vi "S4GUI.vi"(7 "Tab ObsEng":enum32{"Obs", "CCD modes", "Eng"}(tab)) -> ()   [LabVIEW 2018] (continued)
                n2324 = call "Write Exposure Time.vi"("error in (no error)"=w4861, "Exposure Time"=w4839, "Interface in"=w4872) -> ("error out"=w4840:errorcluster, "Interface out"=w4841:refnum<class "Interface.lvclass">)  [unwired: 7 in]
                n2325 = case shown="Default" w4838 {
                  tunnel: w4841 -> [w4887 w4892]
                  tunnel: [w4887 w4891] -> w4837
                  tunnel: [w4886 w4890] -> w4836
                  tunnel: w4840 -> [w4886 w4889]
                  tunnel: w4839 -> [_ w4888]
                  frame "ZERO" {
                  }
                  frame Default {
                    n2326 = call-dynamic "Write prev ExpTime.vi"("error in (no error)"=w4889, "prev ExpTime"=w4888, "Interface in"=w4892) -> ("error out"=w4890:errorcluster, "Interface out"=w4891:refnum<class "Interface.lvclass">)  [unwired: 7 in]
                  }
                }
                n2327 = call-dynamic "Write Suffix.vi"("error in (no error)"=w4836, "Suffix"=w4881, "Interface in"=w4837) -> ("error out"=w4862:errorcluster, "Interface out"=w4873:refnum<class "Interface.lvclass">)  [unwired: 7 in]
                n2328 = call-dynamic "Write ObsType.vi"("error in (no error)"=w4862, "ObsType"=w4856, "Interface in"=w4873) -> ("error out"=w4863:errorcluster, "Interface out"=w4874:refnum<class "Interface.lvclass">)  [unwired: 7 in]
                n2329 = call-dynamic "Write Object.vi"("error in (no error)"=w4863, "Object"=w4855, "Interface in"=w4874) -> ("error out"=w4864:errorcluster, "Interface out"=w4875:refnum<class "Interface.lvclass">)  [unwired: 7 in]
                n2330 = call-dynamic "Write Comments.vi"("error in (no error)"=w4864, "Comments"=w4880, "Interface in"=w4875) -> ("error out"=w4865:errorcluster, "Interface out"=w4876:refnum<class "Interface.lvclass">)  [unwired: 7 in]
                n2331 = local read "Exp ch2"() -> (w4859:u32)
                n2332 = call-dynamic "Write DS9.vi"("error in (no error)"=w4865, "DS9"="F", "Interface in"=w4876) -> ("error out"=w4852:errorcluster, "Interface out"=w4854:refnum<class "Interface.lvclass">)  [unwired: 7 in]
                n2333 = call-dynamic "Write Observer.vi"("error in (no error)"=w4852, "Observer"=w4850, "Interface in"=w4854) -> ("error out"=w4851:errorcluster, "Interface out"=w4853:refnum<class "Interface.lvclass">)  [unwired: 7 in]
                n2334 = call-dynamic "Write # Images.vi"("error in (no error)"=w4851, "# Images"=w4859, "Interface in"=w4853) -> ("error out"=w4866:errorcluster, "Interface out"=w4877:refnum<class "Interface.lvclass">)  [unwired: 7 in]
                n2335 = property on="Exposure Time ch2" class="Slide (strict)"("Scale.Maximum"=w4839, "Scale.Minimum"=0.0 ("Scale.Range:Minimum")) -> ()  [unwired: 2 in, 2 out]
                n2336 = property on="Exposures Done ch2" class="Slide (strict)"("Scale.Maximum"=w4859, "Scale.Minimum"=0.0 ("Scale.Range:Minimum")) -> ()  [unwired: 2 in, 2 out]
                n2337 = call-dynamic "Write Interface.vi"("error in (no error)"=w4866, "Interface.lvclass"=w4877, "Channel in"=w4871) -> ("error out"=w4849:errorcluster, "Channel out"=w4848:refnum<class "Channel.lvclass">)  [unwired: 7 in]
                n2338 = call-dynamic "Write ciclos.vi"("error in (no error)"=w4849, "ciclos"=w4847, "Channel in"=w4848) -> ("error out"=w4844:errorcluster, "Channel out"=w4846:refnum<class "Channel.lvclass">)  [unwired: 7 in]
                n2339 = call-dynamic "Write sequencias.vi"("error in (no error)"=w4844, "sequencias"=w4842, "Channel in"=w4846) -> ("error out"=w4843:errorcluster, "Channel out"=w4845:refnum<class "Channel.lvclass">)  [unwired: 7 in]
                n2340 = call-dynamic "Write Channel.vi"("error in (no error)"=w4843, "Channel.lvclass"=w4845, "Acquisition in"=w4879) -> ("error out"=w4833:errorcluster, "Acquisition out"=w4835:refnum<class "Acquisition.lvclass">)  [unwired: 7 in]
                n2341 = call-dynamic "CalcCubeDuration.vi"("error in (no error)"=w4833, "Acquisition in"=w4835) -> ("error out"=w4832:errorcluster, "Acquisition out"=w4834:refnum<class "Acquisition.lvclass">)  [unwired: 8 in]
                n2342 = call "Write AcquisitionB.vi"("error in (no error)"=w4832, "Acquisition.lvclass"=w4834, "S4ACS_GUI in"=w4878) -> ("error out"=w4882:errorcluster, "S4ACS_GUI out"=w4883:refnum<class "S4GUI.lvclass">)  [unwired: 7 in]
              }
              frame #2 {
                # "object"
                # "suffix"
                # "obsType"
                n2343 = call-dynamic "Read AcquisitionC.vi"("error in (no error)"=w4945, "S4ACS_GUI in"=w4946) -> ("error out"=w4935:errorcluster, "Acquisition.lvclass"=w4934:refnum<class "Acquisition.lvclass">, "S4ACS_GUI out"=w4924:refnum<class "S4GUI.lvclass">)  [unwired: 7 in]
                n2344 = call-dynamic "Read Channel.vi"("error in (no error)"=w4935, "Acquisition in"=w4934) -> ("error out"=w4932:errorcluster, "Channel.lvclass"=w4933:refnum<class "Channel.lvclass">, "Acquisition out"=w4923:refnum<class "Acquisition.lvclass">)  [unwired: 7 in]
                n2345 = local read "Exptime ch3"() -> (w4900:dbl)
                n2346 = call-dynamic "Read Interface.vi"("error in (no error)"=w4932, "Channel in"=w4933) -> ("error out"=w4941:errorcluster, "Interface.lvclass"=w4930:refnum<class "Interface.lvclass">, "Channel out"=w4931:refnum<class "Channel.lvclass">)  [unwired: 7 in]
                n2347 = call "Write Exposure Time.vi"("error in (no error)"=w4941, "Exposure Time"=w4900, "Interface in"=w4930) -> ("error out"=w4901:errorcluster, "Interface out"=w4902:refnum<class "Interface.lvclass">)  [unwired: 7 in]
                n2348 = case shown="\"ZERO\"" w4899 {
                  tunnel: w4902 -> [w4948 w4953]
                  tunnel: [w4948 w4952] -> w4898
                  tunnel: [w4947 w4951] -> w4897
                  tunnel: w4901 -> [w4947 w4950]
                  tunnel: w4900 -> [_ w4949]
                  frame "ZERO" {
                  }
                  frame Default {
                    n2349 = call-dynamic "Write prev ExpTime.vi"("error in (no error)"=w4950, "prev ExpTime"=w4949, "Interface in"=w4953) -> ("error out"=w4951:errorcluster, "Interface out"=w4952:refnum<class "Interface.lvclass">)  [unwired: 7 in]
                  }
                }
                n2350 = call-dynamic "Write Suffix.vi"("error in (no error)"=w4897, "Suffix"=w4942, "Interface in"=w4898) -> ("error out"=w4940:errorcluster, "Interface out"=w4929:refnum<class "Interface.lvclass">)  [unwired: 7 in]
                n2351 = call-dynamic "Write ObsType.vi"("error in (no error)"=w4940, "ObsType"=w4917, "Interface in"=w4929) -> ("error out"=w4939:errorcluster, "Interface out"=w4928:refnum<class "Interface.lvclass">)  [unwired: 7 in]
                n2352 = call-dynamic "Write Object.vi"("error in (no error)"=w4939, "Object"=w4916, "Interface in"=w4928) -> ("error out"=w4938:errorcluster, "Interface out"=w4927:refnum<class "Interface.lvclass">)  [unwired: 7 in]
                n2353 = call-dynamic "Write Comments.vi"("error in (no error)"=w4938, "Comments"=w4918, "Interface in"=w4927) -> ("error out"=w4937:errorcluster, "Interface out"=w4926:refnum<class "Interface.lvclass">)  [unwired: 7 in]
                n2354 = call-dynamic "Write DS9.vi"("error in (no error)"=w4937, "DS9"="F", "Interface in"=w4926) -> ("error out"=w4913:errorcluster, "Interface out"=w4915:refnum<class "Interface.lvclass">)  [unwired: 7 in]
                n2355 = local read "Exp ch3"() -> (w4921:u32)
                n2356 = property on="Exposure Time ch3" class="Slide (strict)"("Scale.Maximum"=w4900, "Scale.Minimum"=0.0 ("Scale.Range:Minimum")) -> ()  [unwired: 2 in, 2 out]
                n2357 = call-dynamic "Write Observer.vi"("error in (no error)"=w4913, "Observer"=w4911, "Interface in"=w4915) -> ("error out"=w4912:errorcluster, "Interface out"=w4914:refnum<class "Interface.lvclass">)  [unwired: 7 in]
                n2358 = property on="Exposures Done ch3" class="Slide (strict)"("Scale.Maximum"=w4921, "Scale.Minimum"=0.0 ("Scale.Range:Minimum")) -> ()  [unwired: 2 in, 2 out]
                n2359 = call-dynamic "Write # Images.vi"("error in (no error)"=w4912, "# Images"=w4921, "Interface in"=w4914) -> ("error out"=w4936:errorcluster, "Interface out"=w4925:refnum<class "Interface.lvclass">)  [unwired: 7 in]
                n2360 = call-dynamic "Write Interface.vi"("error in (no error)"=w4936, "Interface.lvclass"=w4925, "Channel in"=w4931) -> ("error out"=w4910:errorcluster, "Channel out"=w4909:refnum<class "Channel.lvclass">)  [unwired: 7 in]
                n2361 = call-dynamic "Write ciclos.vi"("error in (no error)"=w4910, "ciclos"=w4908, "Channel in"=w4909) -> ("error out"=w4905:errorcluster, "Channel out"=w4907:refnum<class "Channel.lvclass">)  [unwired: 7 in]
                n2362 = call-dynamic "Write sequencias.vi"("error in (no error)"=w4905, "sequencias"=w4903, "Channel in"=w4907) -> ("error out"=w4904:errorcluster, "Channel out"=w4906:refnum<class "Channel.lvclass">)  [unwired: 7 in]
                n2363 = call-dynamic "Write Channel.vi"("error in (no error)"=w4904, "Channel.lvclass"=w4906, "Acquisition in"=w4923) -> ("error out"=w4894:errorcluster, "Acquisition out"=w4896:refnum<class "Acquisition.lvclass">)  [unwired: 7 in]
                n2364 = call-dynamic "CalcCubeDuration.vi"("error in (no error)"=w4894, "Acquisition in"=w4896) -> ("error out"=w4893:errorcluster, "Acquisition out"=w4895:refnum<class "Acquisition.lvclass">)  [unwired: 8 in]
                n2365 = call-dynamic "Write AcquisitionC.vi"("error in (no error)"=w4893, "Acquisition.lvclass"=w4895, "S4ACS_GUI in"=w4924) -> ("error out"=w4943:errorcluster, "S4ACS_GUI out"=w4944:refnum<class "S4GUI.lvclass">)  [unwired: 7 in]
              }
              frame #3 {
                # "object"
                # "suffix"
                # "obsType"
                n2366 = call-dynamic "Read AcquisitionD.vi"("error in (no error)"=w5006, "S4ACS_GUI in"=w5007) -> ("error out"=w4996:errorcluster, "Acquisition.lvclass"=w4995:refnum<class "Acquisition.lvclass">, "S4ACS_GUI out"=w4985:refnum<class "S4GUI.lvclass">)  [unwired: 7 in]
                n2367 = local read "Exptime ch4"() -> (w4959:dbl)
                n2368 = call-dynamic "Read Channel.vi"("error in (no error)"=w4996, "Acquisition in"=w4995) -> ("error out"=w4993:errorcluster, "Channel.lvclass"=w4994:refnum<class "Channel.lvclass">, "Acquisition out"=w4984:refnum<class "Acquisition.lvclass">)  [unwired: 7 in]
                n2369 = call-dynamic "Read Interface.vi"("error in (no error)"=w4993, "Channel in"=w4994) -> ("error out"=w5002:errorcluster, "Interface.lvclass"=w4991:refnum<class "Interface.lvclass">, "Channel out"=w4992:refnum<class "Channel.lvclass">)  [unwired: 7 in]
                n2370 = call "Write Exposure Time.vi"("error in (no error)"=w5002, "Exposure Time"=w4959, "Interface in"=w4991) -> ("error out"=w4961:errorcluster, "Interface out"=w4963:refnum<class "Interface.lvclass">)  [unwired: 7 in]
                n2371 = case shown="Default" w4958 {
                  tunnel: w4963 -> [w5009 w5014]
                  tunnel: [w5009 w5013] -> w4962
                  tunnel: [w5008 w5012] -> w4960
                  tunnel: w4961 -> [w5008 w5011]
                  tunnel: w4959 -> [_ w5010]
                  frame "ZERO" {
                  }
                  frame Default {
                    n2372 = call-dynamic "Write prev ExpTime.vi"("error in (no error)"=w5011, "prev ExpTime"=w5010, "Interface in"=w5014) -> ("error out"=w5012:errorcluster, "Interface out"=w5013:refnum<class "Interface.lvclass">)  [unwired: 7 in]
                  }
                }
                n2373 = call-dynamic "Write Suffix.vi"("error in (no error)"=w4960, "Suffix"=w5003, "Interface in"=w4962) -> ("error out"=w5001:errorcluster, "Interface out"=w4990:refnum<class "Interface.lvclass">)  [unwired: 7 in]
                n2374 = call-dynamic "Write ObsType.vi"("error in (no error)"=w5001, "ObsType"=w4978, "Interface in"=w4990) -> ("error out"=w5000:errorcluster, "Interface out"=w4989:refnum<class "Interface.lvclass">)  [unwired: 7 in]
                n2375 = call-dynamic "Write Object.vi"("error in (no error)"=w5000, "Object"=w4977, "Interface in"=w4989) -> ("error out"=w4999:errorcluster, "Interface out"=w4988:refnum<class "Interface.lvclass">)  [unwired: 7 in]
                n2376 = call-dynamic "Write Comments.vi"("error in (no error)"=w4999, "Comments"=w4979, "Interface in"=w4988) -> ("error out"=w4998:errorcluster, "Interface out"=w4987:refnum<class "Interface.lvclass">)  [unwired: 7 in]
                n2377 = call-dynamic "Write DS9.vi"("error in (no error)"=w4998, "DS9"="F", "Interface in"=w4987) -> ("error out"=w4974:errorcluster, "Interface out"=w4976:refnum<class "Interface.lvclass">)  [unwired: 7 in]
                n2378 = property on="Exposure Time ch4" class="Slide (strict)"("Scale.Maximum"=w4959, "Scale.Minimum"=0.0 ("Scale.Range:Minimum")) -> ()  [unwired: 2 in, 2 out]
                n2379 = local read "Exp ch4"() -> (w4982:u32)
                n2380 = call-dynamic "Write Observer.vi"("error in (no error)"=w4974, "Observer"=w4972, "Interface in"=w4976) -> ("error out"=w4973:errorcluster, "Interface out"=w4975:refnum<class "Interface.lvclass">)  [unwired: 7 in]
                n2381 = property on="Exposures Done ch4" class="Slide (strict)"("Scale.Maximum"=w4982, "Scale.Minimum"=0.0 ("Scale.Range:Minimum")) -> ()  [unwired: 2 in, 2 out]
                n2382 = call-dynamic "Write # Images.vi"("error in (no error)"=w4973, "# Images"=w4982, "Interface in"=w4975) -> ("error out"=w4997:errorcluster, "Interface out"=w4986:refnum<class "Interface.lvclass">)  [unwired: 7 in]
                n2383 = call-dynamic "Write Interface.vi"("error in (no error)"=w4997, "Interface.lvclass"=w4986, "Channel in"=w4992) -> ("error out"=w4971:errorcluster, "Channel out"=w4970:refnum<class "Channel.lvclass">)  [unwired: 7 in]
                n2384 = call-dynamic "Write ciclos.vi"("error in (no error)"=w4971, "ciclos"=w4969, "Channel in"=w4970) -> ("error out"=w4967:errorcluster, "Channel out"=w4968:refnum<class "Channel.lvclass">)  [unwired: 7 in]
                n2385 = call-dynamic "Write sequencias.vi"("error in (no error)"=w4967, "sequencias"=w4964, "Channel in"=w4968) -> ("error out"=w4966:errorcluster, "Channel out"=w4965:refnum<class "Channel.lvclass">)  [unwired: 7 in]
                n2386 = call-dynamic "Write Channel.vi"("error in (no error)"=w4966, "Channel.lvclass"=w4965, "Acquisition in"=w4984) -> ("error out"=w4955:errorcluster, "Acquisition out"=w4957:refnum<class "Acquisition.lvclass">)  [unwired: 7 in]
                n2387 = call-dynamic "CalcCubeDuration.vi"("error in (no error)"=w4955, "Acquisition in"=w4957) -> ("error out"=w4954:errorcluster, "Acquisition out"=w4956:refnum<class "Acquisition.lvclass">)  [unwired: 8 in]
                n2388 = call-dynamic "Write AcquisitionD.vi"("error in (no error)"=w4954, "Acquisition.lvclass"=w4956, "S4ACS_GUI in"=w4985) -> ("error out"=w5004:errorcluster, "S4ACS_GUI out"=w5005:refnum<class "S4GUI.lvclass">)  [unwired: 7 in]
              }
            }
            n2389 = call-dynamic "Write sequencias.vi"("error in (no error)"=w4730, "sequencias"=w4726, "S4GUI in"=w4728) -> ("error out"=w4729:errorcluster, "S4GUI out"=w4727:refnum<class "S4GUI.lvclass">)  [unwired: 7 in]
            n2390 = call-dynamic "Write ciclos.vi"("error in (no error)"=w4729, "ciclos"=w4731, "S4ACS_GUI in"=w4727) -> ("error out"=w4733:errorcluster, "S4ACS_GUI out"=w4735:refnum<class "S4GUI.lvclass">)  [unwired: 7 in]
            n2391 = property on="#Cycles Done" class="Slide (strict)"("Scale.Maximum"=w4731, "Scale.Minimum"=0.0 ("Scale.Range:Minor Increment")) -> ()  [unwired: 2 in, 2 out]
            n2392 = call-dynamic "Write TotalCiclos.vi"("error in (no error)"=w4733, "TotalCiclos"=w4731, "S4GUI in"=w4735) -> ("error out"=w4732:errorcluster, "S4GUI out"=w4734:refnum<class "S4GUI.lvclass">)  [unwired: 7 in]
          }
        }
        n2393 = call-dynamic "Write User Event.vi"("error in (no error)"=w4567, "User Event"=w4564, "S4GUI in"=w4568) -> ("error out"=w4566:errorcluster, "S4GUI out"=w4565:refnum<class "S4GUI.lvclass">)  [unwired: 7 in]
        n2394 = property on="Pause SM" class="Bool"(error in=w4566, "DisabledEnum"=T12."Enabled" ("Disabled")) -> (error out=w4585:errorcluster)  [unwired: 1 in, 1 out]
      }
      event "# Cycles": Value Change {
        w5015 = 0.0 ("Scale.Range:Minor Increment")
        n2395 = event-data() -> ("NewVal"=w5016:u32)  [unwired: 1 in]
        n2396 = call-dynamic "Write ciclos.vi"("error in (no error)"=w5019, "ciclos"=w5016, "S4ACS_GUI in"=w5020) -> ("error out"=w5018:errorcluster, "S4ACS_GUI out"=w5017:refnum<class "S4GUI.lvclass">)  [unwired: 7 in]
        n2397 = property on="#Cycles Done" class="Slide (strict)"("Scale.Maximum"=w5016, "Scale.Minimum"=w5015) -> ()  [unwired: 2 in, 2 out]
        n2398 = property on="Cycles Done ch2" class="Slide (strict)"("Scale.Maximum"=w5016, "Scale.Minimum"=w5015) -> ()  [unwired: 2 in, 2 out]
        n2399 = property on="Cycles Done ch4" class="Slide (strict)"("Scale.Maximum"=w5016, "Scale.Minimum"=w5015) -> ()  [unwired: 2 in, 2 out]
        n2400 = property on="Cycles Done ch1" class="Slide (strict)"("Scale.Maximum"=w5016, "Scale.Minimum"=w5015) -> ()  [unwired: 2 in, 2 out]
        n2401 = property on="Cycles Done ch3" class="Slide (strict)"("Scale.Maximum"=w5016, "Scale.Minimum"=w5015) -> ()  [unwired: 2 in, 2 out]
      }
      event "AllConfig": Value Change {
        n2402 = event-data() -> ()  [unwired: 1 in, 6 out]
        n2403 = call "Read Instrument.lvclass.vi"("error in (no error)"=w5025, "S4ACS_GUI in"=w5026) -> ("error out"=w5105:errorcluster, "Instrument.lvclass"=w5072:refnum<class "Instrument.lvclass">, "S4ACS_GUI out"=w5103:refnum<class "S4GUI.lvclass">)  [unwired: 7 in]
        n2404 = call "Read ASEL.vi"("error in (no error)"=w5105, "Instrument in"=w5072) -> ("error out"=w5097:errorcluster, "Opt_Selector.lvclass"=w5096:refnum<class "Opt_Selector.lvclass">, "Instrument out"=w5104:refnum<class "Instrument.lvclass">)  [unwired: 7 in]
        n2405 = call-dynamic "Read State Machine.vi"("error in (no error)"=w5097, "Device in"=w5096) -> ("error out"=w5100:errorcluster, "State Machine.lvclass"=w5102:refnum<class "State Machine.lvclass">, "Device out"=w5094:refnum<class "Opt_Selector.lvclass">)  [unwired: 7 in]
        n2406 = call "Next State.vi"("error in (no error)"=w5100, "New_State"=1, "State Machine in"=w5102) -> ("error out"=w5099:errorcluster, "State Machine out"=w5098:refnum<class "State Machine.lvclass">)  [unwired: 7 in]
        n2407 = call-dynamic "Write State Machine.vi"("error in (no error)"=w5099, "State Machine.lvclass"=w5098, "Device in"=w5094) -> ("error out"=w5093:errorcluster, "Device out"=w5095:refnum<class "Opt_Selector.lvclass">)  [unwired: 7 in]
        n2408 = call "Write ASEL.vi"("error in (no error)"=w5093, "Opt_Selector.lvclass"=w5095, "Instrument in"=w5104) -> ("error out"=w5055:errorcluster, "Instrument out"=w5071:refnum<class "Instrument.lvclass">)  [unwired: 7 in]
        n2409 = call "Read CALW.vi"("error in (no error)"=w5055, "Instrument in"=w5071) -> ("error out"=w5088:errorcluster, "Opt_Selector.lvclass"=w5089:refnum<class "Opt_Selector.lvclass">, "Instrument out"=w5070:refnum<class "Instrument.lvclass">)  [unwired: 7 in]
        n2410 = call-dynamic "Read State Machine.vi"("error in (no error)"=w5088, "Device in"=w5089) -> ("error out"=w5085:errorcluster, "State Machine.lvclass"=w5083:refnum<class "State Machine.lvclass">, "Device out"=w5091:refnum<class "Opt_Selector.lvclass">)  [unwired: 7 in]
        n2411 = call "Next State.vi"("error in (no error)"=w5085, "New_State"=1, "State Machine in"=w5083) -> ("error out"=w5086:errorcluster, "State Machine out"=w5087:refnum<class "State Machine.lvclass">)  [unwired: 7 in]
        n2412 = call-dynamic "Write State Machine.vi"("error in (no error)"=w5086, "State Machine.lvclass"=w5087, "Device in"=w5091) -> ("error out"=w5092:errorcluster, "Device out"=w5090:refnum<class "Opt_Selector.lvclass">)  [unwired: 7 in]
        n2413 = call "Write CALW.vi"("error in (no error)"=w5092, "Opt_Selector.lvclass"=w5090, "Instrument in"=w5070) -> ("error out"=w5054:errorcluster, "Instrument out"=w5069:refnum<class "Instrument.lvclass">)  [unwired: 7 in]
        n2414 = call "Read WPSEL.vi"("error in (no error)"=w5054, "Instrument in"=w5069) -> ("error out"=w5077:errorcluster, "Opt_Selector.lvclass"=w5076:refnum<class "Opt_Selector.lvclass">, "Instrument out"=w5068:refnum<class "Instrument.lvclass">)  [unwired: 7 in]
        n2415 = call-dynamic "Read State Machine.vi"("error in (no error)"=w5077, "Device in"=w5076) -> ("error out"=w5080:errorcluster, "State Machine.lvclass"=w5082:refnum<class "State Machine.lvclass">, "Device out"=w5074:refnum<class "Opt_Selector.lvclass">)  [unwired: 7 in]
        n2416 = call "Next State.vi"("error in (no error)"=w5080, "New_State"=1, "State Machine in"=w5082) -> ("error out"=w5079:errorcluster, "State Machine out"=w5078:refnum<class "State Machine.lvclass">)  [unwired: 7 in]
        n2417 = call-dynamic "Write State Machine.vi"("error in (no error)"=w5079, "State Machine.lvclass"=w5078, "Device in"=w5074) -> ("error out"=w5073:errorcluster, "Device out"=w5075:refnum<class "Opt_Selector.lvclass">)  [unwired: 7 in]
        n2418 = call "Write WPSEL.vi"("error in (no error)"=w5073, "Opt_Selector.lvclass"=w5075, "Instrument in"=w5068) -> ("error out"=w5053:errorcluster, "Instrument out"=w5057:refnum<class "Instrument.lvclass">)  [unwired: 7 in]
        n2419 = call "Read WPROT.vi"("error in (no error)"=w5053, "Instrument in"=w5057) -> ("error out"=w5063:errorcluster, "Opt_Selector.lvclass"=w5064:refnum<class "Opt_Selector.lvclass">, "Instrument out"=w5056:refnum<class "Instrument.lvclass">)  [unwired: 7 in]
        n2420 = call-dynamic "Read State Machine.vi"("error in (no error)"=w5063, "Device in"=w5064) -> ("error out"=w5060:errorcluster, "State Machine.lvclass"=w5058:refnum<class "State Machine.lvclass">, "Device out"=w5066:refnum<class "Opt_Selector.lvclass">)  [unwired: 7 in]
        n2421 = call "Next State.vi"("error in (no error)"=w5060, "New_State"=1, "State Machine in"=w5058) -> ("error out"=w5061:errorcluster, "State Machine out"=w5062:refnum<class "State Machine.lvclass">)  [unwired: 7 in]
        n2422 = call-dynamic "Write State Machine.vi"("error in (no error)"=w5061, "State Machine.lvclass"=w5062, "Device in"=w5066) -> ("error out"=w5067:errorcluster, "Device out"=w5065:refnum<class "Opt_Selector.lvclass">)  [unwired: 7 in]
        n2423 = call "Write WPROT.vi"("error in (no error)"=w5067, "Opt_Selector.lvclass"=w5065, "Instrument in"=w5056) -> ("error out"=w5029:errorcluster, "Instrument out"=w5030:refnum<class "Instrument.lvclass">)  [unwired: 7 in]
        n2424 = call "Read GMIR.vi"("error in (no error)"=w5029, "Instrument in"=w5030) -> ("error out"=w5048:errorcluster, "Opt_Continuous.lvclass"=w5049:refnum<class "Opt_Continuous.lvclass">, "Instrument out"=w5042:refnum<class "Instrument.lvclass">)  [unwired: 7 in]
        n2425 = call-dynamic "Read State Machine.vi"("error in (no error)"=w5048, "Device in"=w5049) -> ("error out"=w5045:errorcluster, "State Machine.lvclass"=w5043:refnum<class "State Machine.lvclass">, "Device out"=w5051:refnum<class "Opt_Continuous.lvclass">)  [unwired: 7 in]
        n2426 = call "Next State.vi"("error in (no error)"=w5045, "New_State"=1, "State Machine in"=w5043) -> ("error out"=w5046:errorcluster, "State Machine out"=w5047:refnum<class "State Machine.lvclass">)  [unwired: 7 in]
        n2427 = call-dynamic "Write State Machine.vi"("error in (no error)"=w5046, "State Machine.lvclass"=w5047, "Device in"=w5051) -> ("error out"=w5052:errorcluster, "Device out"=w5050:refnum<class "Opt_Continuous.lvclass">)  [unwired: 7 in]
        n2428 = call "Write GMIR.vi"("error in (no error)"=w5052, "Opt_Continuous.lvclass"=w5050, "Instrument in"=w5042) -> ("error out"=w5027:errorcluster, "Instrument out"=w5028:refnum<class "Instrument.lvclass">)  [unwired: 7 in]
        n2429 = call "Read GFOC.vi"("error in (no error)"=w5027, "Instrument in"=w5028) -> ("error out"=w5037:errorcluster, "Opt_Continuous.lvclass"=w5038:refnum<class "Opt_Continuous.lvclass">, "Instrument out"=w5031:refnum<class "Instrument.lvclass">)  [unwired: 7 in]
        n2430 = call-dynamic "Read State Machine.vi"("error in (no error)"=w5037, "Device in"=w5038) -> ("error out"=w5034:errorcluster, "State Machine.lvclass"=w5032:refnum<class "State Machine.lvclass">, "Device out"=w5040:refnum<class "Opt_Continuous.lvclass">)  [unwired: 7 in]
        n2431 = call "Next State.vi"("error in (no error)"=w5034, "New_State"=1, "State Machine in"=w5032) -> ("error out"=w5035:errorcluster, "State Machine out"=w5036:refnum<class "State Machine.lvclass">)  [unwired: 7 in]
        n2432 = call-dynamic "Write State Machine.vi"("error in (no error)"=w5035, "State Machine.lvclass"=w5036, "Device in"=w5040) -> ("error out"=w5041:errorcluster, "Device out"=w5039:refnum<class "Opt_Continuous.lvclass">)  [unwired: 7 in]
        n2433 = call "Write GFOC.vi"("error in (no error)"=w5041, "Opt_Continuous.lvclass"=w5039, "Instrument in"=w5031) -> ("error out"=w5023:errorcluster, "Instrument out"=w5024:refnum<class "Instrument.lvclass">)  [unwired: 7 in]
        n2434 = call "Write Instrument.lvclass.vi"("error in (no error)"=w5023, "Instrument.lvclass"=w5024, "S4ACS_GUI in"=w5103) -> ("error out"=w5022:errorcluster, "S4ACS_GUI out"=w5021:refnum<class "S4GUI.lvclass">)  [unwired: 7 in]
      }
      event "Tab Acq Type": Value Change {
        # "Tab for choosing EXPOSURE MODE: Object, Dflat, Sflat, Dark, Zero, Focus"
        n2435 = event-data() -> ("NewVal"=w5139:T1)  [unwired: 1 in]
        n2436 = local read "Observer"() -> (w5137:string)
        n2437 = case shown="\"ZERO\"" w5139 {
          tunnel: ["OBJECT" "FLAT" "FLAT" "DARK" "ZERO" "FOCUS"] -> w5114
          tunnel: [w5210 w5214 w5218 w5222 w5226 w5230] -> w5113
          tunnel: [w5209 w5213 w5217 w5221 w5225 w5229] -> w5138
          tunnel: [w5208 w5212 w5216 w5220 w5224 w5228] -> w5110
          frame "OBJECT", Default {
            n2438 = local read "Object_obj"() -> (w5210:string)
            n2439 = local read "OBJECT Comments"() -> (w5208:string)
            n2440 = local read "object suffix"() -> (w5209:string)
          }
          frame "DFLAT" {
            n2441 = local read "DFLAT Comments"() -> (w5212:string)
            n2442 = local read "Object_dflat"() -> (w5214:string)
            n2443 = local read "dflat suffix"() -> (w5213:string)
          }
          frame "SFLAT" {
            n2444 = local read "SFLAT Comments"() -> (w5216:string)
            n2445 = local read "Object_sflat"() -> (w5218:string)
            n2446 = local read "sflat suffix"() -> (w5217:string)
          }
          frame "DARK" {
            n2447 = local read "Object_dark"() -> (w5222:string)
            n2448 = local read "dark suffix"() -> (w5221:string)
            n2449 = local read "DARK Comments"() -> (w5220:string)
          }
          frame "ZERO" {
            n2450 = local read "ZERO Comments"() -> (w5224:string)
            n2451 = local read "Object_zero"() -> (w5226:string)
            n2452 = local read "zero suffix"() -> (w5225:string)
          }
          frame "FOCUS" {
            n2453 = local read "FOCUS Comments"() -> (w5228:string)
            n2454 = local read "Object_focus"() -> (w5230:string)
            n2455 = local read "focus suffix"() -> (w5229:string)
          }
        }
        n2456 = call-dynamic "Write ExpMode.vi"("error in (no error)"=w5140, "ExpMode"=w5139, "S4GUI in"=w5141) -> ("error out"=w5133:errorcluster, "S4GUI out"=w5132:refnum<class "S4GUI.lvclass">)  [unwired: 7 in]
        n2457 = Concatenate Strings("ACQ TAB SELECTED:" ("User Event"), w5114) -> (w5134:string)
        n2458 = call-dynamic "Write User Event.vi"("error in (no error)"=w5133, "User Event"=w5134, "S4GUI in"=w5132) -> ("error out"=w5117:errorcluster, "S4GUI out"=w5118:refnum<class "S4GUI.lvclass">)  [unwired: 7 in]
        n2459 = call-dynamic "Read Publisher.lvclass.vi"("error in (no error)"=w5117, "S4GUI in"=w5118) -> ("error out"=w5130:errorcluster, "Publisher.lvclass"=w5126:refnum<class "Publisher.lvclass">, "S4GUI out"=w5131:refnum<class "S4GUI.lvclass">)  [unwired: 7 in]
        n2460 = call-dynamic "Write object.vi"("error in (no error)"=w5130, "object"=w5113, "Publisher in"=w5126) -> ("error out"=w5129:errorcluster, "Publisher out"=w5125:refnum<class "Publisher.lvclass">)  [unwired: 7 in]
        n2461 = call-dynamic "Write obstype.vi"("error in (no error)"=w5129, "obstype"=w5114, "Publisher in"=w5125) -> ("error out"=w5128:errorcluster, "Publisher out"=w5124:refnum<class "Publisher.lvclass">)  [unwired: 7 in]
        n2462 = call-dynamic "Write observer.vi"("error in (no error)"=w5128, "observer"=w5112, "Publisher in"=w5124) -> ("error out"=w5127:errorcluster, "Publisher out"=w5123:refnum<class "Publisher.lvclass">)  [unwired: 7 in]
        n2463 = call-dynamic "Write projid.vi"("error in (no error)"=w5127, "projid"=w5111, "Publisher in"=w5123) -> ("error out"=w5120:errorcluster, "Publisher out"=w5119:refnum<class "Publisher.lvclass">)  [unwired: 7 in]
        n2464 = call-dynamic "Write comments.vi"("error in (no error)"=w5120, "comments"=w5110, "Publisher in"=w5119) -> ("error out"=w5122:errorcluster, "Publisher out"=w5121:refnum<class "Publisher.lvclass">)  [unwired: 7 in]
        n2465 = call-dynamic "Write Publisher.lvclass.vi"("error in (no error)"=w5122, "Publisher.lvclass"=w5121, "S4GUI in"=w5131) -> ("error out"=w5116:errorcluster, "S4GUI out"=w5115:refnum<class "S4GUI.lvclass">)  [unwired: 7 in]
        n2466 = call-dynamic "Read AcquisitionA.vi"("error in (no error)"=w5116, "S4ACS_GUI in"=w5115) -> ("error out"=w5148:errorcluster, "Acquisition.lvclass"=w5149:refnum<class "Acquisition.lvclass">, "S4ACS_GUI out"=w5168:refnum<class "S4GUI.lvclass">)  [unwired: 7 in]
        n2467 = call-dynamic "Read AcquisitionC.vi"("error in (no error)"=w5117, "S4ACS_GUI in"=w5118) -> ("error out"=w5144:errorcluster, "Acquisition.lvclass"=w5145:refnum<class "Acquisition.lvclass">)  [unwired: 7 in, 1 out]
        n2468 = call "Read AcquisitionB.vi"("error in (no error)"=w5117, "S4ACS_GUI in"=w5118) -> ("error out"=w5146:errorcluster, "Acquisition.lvclass"=w5147:refnum<class "Acquisition.lvclass">)  [unwired: 7 in, 1 out]
        n2469 = call-dynamic "Read AcquisitionD.vi"("error in (no error)"=w5117, "S4ACS_GUI in"=w5118) -> ("error out"=w5142:errorcluster, "Acquisition.lvclass"=w5143:refnum<class "Acquisition.lvclass">)  [unwired: 7 in, 1 out]
        n2470 = To Lower Case(string=w5138) -> (all lower case string=w5136:string)
        n2471 = case shown="\"DARK\"" w5139 {
          tunnel: [w5265 w5642 w6047] -> w5167
          tunnel: [w5264 w5641 w6046] -> w5166
          tunnel: [w5263 w5640 w6045] -> w5164
          tunnel: [w5262 w5639 w6044] -> w5163
          tunnel: [w5261 w5638 w6043] -> w5153
          tunnel: [w5260 w5637 w6042] -> w5152
          tunnel: [w5259 w5636 w6041] -> w5151
          tunnel: [w5258 w5635 w6040] -> w5150
          tunnel: w5149 -> [w5257 w5634 w6039]
          tunnel: w5148 -> [w5256 w5633 w6038]
          tunnel: w5147 -> [w5242 w5620 w6025]
          tunnel: w5146 -> [w5241 w5619 w6024]
          tunnel: w5145 -> [w5240 w5618 w6023]
          tunnel: w5144 -> [w5239 w5617 w6022]
          tunnel: w5143 -> [w5238 w5616 w6021]
          tunnel: w5142 -> [w5237 w5615 w6020]
          tunnel: w5113 -> [w5234 w5614 w6019]
          tunnel: w5110 -> [w5235 w5613 w6018]
          tunnel: w5137 -> [w5236 w5612 w6017]
          tunnel: w5136 -> [w5233 w5611 w6016]
          tunnel: w5114 -> [w5232 w5610 w6015]
          frame "ZERO" {
            w5255 = 1e-05 ("Exptime ch1")
            # "ZERO: EXPTIME=1E-5 (mandatory), shutter automatically closed, save current FRAME_TRANSFER (prev_FT) and reset FRAME_TRANSFER."
            n2472 = call "Read connection.vi"("error in (no error)"=w5239, "Server in"=w5240) -> ("error out"=w5247:errorcluster, "connection"=w5246:bool, "Server out"=w5248:refnum<class "Acquisition.lvclass">)  [unwired: 7 in]
            n2473 = call "Read connection.vi"("error in (no error)"=w5241, "Server in"=w5242) -> ("error out"=w5250:errorcluster, "connection"=w5249:bool, "Server out"=w5251:refnum<class "Acquisition.lvclass">)  [unwired: 7 in]
            n2474 = call "Read connection.vi"("error in (no error)"=w5256, "Server in"=w5257) -> ("error out"=w5253:errorcluster, "connection"=w5252:bool, "Server out"=w5254:refnum<class "Acquisition.lvclass">)  [unwired: 7 in]
            n2475 = call "Read connection.vi"("error in (no error)"=w5237, "Server in"=w5238) -> ("error out"=w5244:errorcluster, "connection"=w5243:bool, "Server out"=w5245:refnum<class "Acquisition.lvclass">)  [unwired: 7 in]
            n2476 = case shown="True" w5249 {
              tunnel: w5251 -> [w5439 w5498]
              tunnel: w5250 -> [w5438 w5497]
              tunnel: [w5439 w5496] -> w5263
              tunnel: [w5438 w5495] -> w5262
              tunnel: w5236 -> [_ w5474]
              tunnel: w5235 -> [_ w5473]
              tunnel: w5234 -> [_ w5472]
              tunnel: w5233 -> [_ w5470]
              tunnel: w5232 -> [_ w5469]
              frame False {
              }
              frame True {
                # "nome do arquivo .cfg"
                # "seção no arquivo .cfg"
                n2477 = call-dynamic "Read Channel.vi"("error in (no error)"=w5497, "Acquisition in"=w5498) -> ("error out"=w5501:errorcluster, "Channel.lvclass"=w5500:refnum<class "Channel.lvclass">, "Acquisition out"=w5499:refnum<class "Acquisition.lvclass">)  [unwired: 7 in]
                n2478 = call-dynamic "Read Interface.vi"("error in (no error)"=w5501, "Channel in"=w5500) -> ("error out"=w5466:errorcluster, "Interface.lvclass"=w5467:refnum<class "Interface.lvclass">, "Channel out"=w5461:refnum<class "Channel.lvclass">)  [unwired: 7 in]
                n2479 = call-dynamic "Write restoreExpTime.vi"("error in (no error)"=w5466, "restoreExpTime"=TRUE, "Interface in"=w5467) -> ("error out"=w5463:errorcluster, "Interface out"=w5465:refnum<class "Interface.lvclass">)  [unwired: 7 in]
                n2480 = call-dynamic "Read target cluster.vi"("error in (no error)"=w5463, "Channel in"=w5461) -> ("error out"=w5462:errorcluster, "target cluster"=w5464:T30, "Channel out"=w5457:refnum<class "Channel.lvclass">)  [unwired: 7 in]
                n2481 = stacked-sequence {
                  tunnel: [_ w5522] -> w5460
                  tunnel: w5464 -> [_ w5521]
                  tunnel: w5464 -> [w5519 _]
                  tunnel: [w5518 _] -> w5471
                  frame #0 {
                    n2482 = Unbundle By Name(w5519) -> ("FRAME_TRANSFER"=w5518:bool)
                  }
                  frame #1 {
                    # "closed"
                    n2483 = Bundle By Name(cluster=w5521, "SHUTTER_MODE"=u8 2, "FRAME_TRANSFER"=FALSE) -> (w5522:T30)
                  }
                }
                n2484 = call-dynamic "Write PREV_FT.vi"("error in (no error)"=w5462, "PREV_FT"=w5471, "Interface in"=w5465) -> ("error out"=w5459:errorcluster, "Interface out"=w5455:refnum<class "Interface.lvclass">)  [unwired: 7 in]
                n2485 = call-dynamic "Write target cluster.vi"("error in (no error)"=w5459, "target cluster"=w5460, "Channel in"=w5457) -> ("error out"=w5458:errorcluster, "Channel out"=w5456:refnum<class "Channel.lvclass">)  [unwired: 7 in]
                n2486 = Flatten To String(anything=w5460, error in (no error)=w5458) -> (data string=w5502:string, error out=w5503:errorcluster)  [unwired: 2 in, 1 out]
                n2487 = call "Write flatted cluster.vi"("error in (no error)"=w5503, "flatted cluster"=w5502, "Interface in"=w5455) -> ("error out"=w5505:errorcluster, "Interface out"=w5504:refnum<class "Interface.lvclass">)  [unwired: 7 in]
                n2488 = call-dynamic "Write Interface.vi"("error in (no error)"=w5505, "Interface.lvclass"=w5504, "Channel in"=w5456) -> ("error out"=w5509:errorcluster, "Channel out"=w5510:refnum<class "Channel.lvclass">)  [unwired: 7 in]
                n2489 = call "Write section_name.vi"("error in (no error)"=w5509, "section_name"="CCD_ACS2", "Channel in"=w5510) -> ("error out"=w5508:errorcluster, "Channel out"=w5513:refnum<class "Channel.lvclass">)  [unwired: 7 in]
                n2490 = call-dynamic "save config.vi"("error in (no error)"=w5508, "file config"="lastsaved.cfg", "Channel in"=w5513) -> ("error out"=w5477:errorcluster, "Channel out"=w5478:refnum<class "Channel.lvclass">)  [unwired: 7 in]
                n2491 = local read "Filter2"() -> (w5479:u8)
                n2492 = call-dynamic "Write Filter.vi"("error in (no error)"=w5477, "Filter"=w5479, "Channel in"=w5478) -> ("error out"=w5486:errorcluster, "Channel out"=w5487:refnum<class "Channel.lvclass">)  [unwired: 7 in]
                n2493 = call-dynamic "Read Interface.vi"("error in (no error)"=w5486, "Channel in"=w5487) -> ("error out"=w5484:errorcluster, "Interface.lvclass"=w5489:refnum<class "Interface.lvclass">, "Channel out"=w5488:refnum<class "Channel.lvclass">)  [unwired: 7 in]
                n2494 = call-dynamic "Write Suffix.vi"("error in (no error)"=w5484, "Suffix"=w5470, "Interface in"=w5489) -> ("error out"=w5480:errorcluster, "Interface out"=w5490:refnum<class "Interface.lvclass">)  [unwired: 7 in]
                n2495 = call-dynamic "Write ObsType.vi"("error in (no error)"=w5480, "ObsType"=w5469, "Interface in"=w5490) -> ("error out"=w5481:errorcluster, "Interface out"=w5491:refnum<class "Interface.lvclass">)  [unwired: 7 in]
                n2496 = call-dynamic "Write Object.vi"("error in (no error)"=w5481, "Object"=w5472, "Interface in"=w5491) -> ("error out"=w5482:errorcluster, "Interface out"=w5492:refnum<class "Interface.lvclass">)  [unwired: 7 in]
                n2497 = call-dynamic "Write Comments.vi"("error in (no error)"=w5482, "Comments"=w5473, "Interface in"=w5492) -> ("error out"=w5483:errorcluster, "Interface out"=w5493:refnum<class "Interface.lvclass">)  [unwired: 7 in]
                n2498 = call-dynamic "Write Observer.vi"("error in (no error)"=w5483, "Observer"=w5474, "Interface in"=w5493) -> ("error out"=w5485:errorcluster, "Interface out"=w5494:refnum<class "Interface.lvclass">)  [unwired: 7 in]
                n2499 = call-dynamic "Write Interface.vi"("error in (no error)"=w5485, "Interface.lvclass"=w5494, "Channel in"=w5488) -> ("error out"=w5476:errorcluster, "Channel out"=w5475:refnum<class "Channel.lvclass">)  [unwired: 7 in]
                n2500 = call-dynamic "Read State Machine.vi"("error in (no error)"=w5476, "Device in"=w5475) -> ("error out"=w5441:errorcluster, "State Machine.lvclass"=w5443:refnum<class "State Machine.lvclass">, "Device out"=w5514:refnum<class "Channel.lvclass">)  [unwired: 7 in]
                n2501 = call-dynamic "Read ref StatesQueue.vi"("error in (no error)"=w5441, "State Machine in"=w5443) -> ("error out"=w5448:errorcluster, "ref StatesQueue"=w5447:refnum<queue>, "State Machine out"=w5444:refnum<class "State Machine.lvclass">)  [unwired: 7 in]
                n2502 = Flush Queue(queue=w5447, error in (no error)=w5448) -> (queue out=w5449:refnum<queue>, error out=w5453:errorcluster)  [unwired: 1 out]
                n2503 = Enqueue Element(queue=w5449, element=u32 300 ("State"), error in (no error)=w5453) -> (queue out=w5450:refnum<queue>, error out=w5454:errorcluster)  [unwired: 1 in, 1 out]
                n2504 = Enqueue Element(queue=w5450, element=u32 60 ("State"), error in (no error)=w5454) -> (queue out=w5451:refnum<queue>, error out=w5452:errorcluster)  [unwired: 1 in, 1 out]
                n2505 = call-dynamic "Write ref StatesQueue.vi"("error in (no error)"=w5452, "ref StatesQueue"=w5451, "State Machine in"=w5444) -> ("error out"=w5440:errorcluster, "State Machine out"=w5442:refnum<class "State Machine.lvclass">)  [unwired: 7 in]
                n2506 = call-dynamic "Write State.vi"("error in (no error)"=w5440, "State"=0, "State Machine in"=w5442) -> ("error out"=w5506:errorcluster, "State Machine out"=w5515:refnum<class "State Machine.lvclass">)  [unwired: 7 in]
                n2507 = call-dynamic "Write State Machine.vi"("error in (no error)"=w5506, "State Machine.lvclass"=w5515, "Device in"=w5514) -> ("error out"=w5517:errorcluster, "Device out"=w5516:refnum<class "Channel.lvclass">)  [unwired: 7 in]
                n2508 = call-dynamic "Write Channel.vi"("error in (no error)"=w5517, "Channel.lvclass"=w5516, "Acquisition in"=w5499) -> ("error out"=w5495:errorcluster, "Acquisition out"=w5496:refnum<class "Acquisition.lvclass">)  [unwired: 7 in]
              }
            }
            n2509 = case shown="True" w5252 {
              tunnel: [w5524 w5600] -> w5264
              tunnel: [w5525 w5599] -> w5265
              tunnel: w5254 -> [w5525 w5582]
              tunnel: w5253 -> [w5524 w5581]
              tunnel: w5236 -> [_ w5560]
              tunnel: w5235 -> [_ w5559]
              tunnel: w5234 -> [_ w5558]
              tunnel: w5233 -> [_ w5556]
              tunnel: w5232 -> [_ w5555]
              frame False {
              }
              frame True {
                # "nome do arquivo .cfg"
                # "seção no arquivo .cfg"
                n2510 = call-dynamic "Read Channel.vi"("error in (no error)"=w5581, "Acquisition in"=w5582) -> ("error out"=w5601:errorcluster, "Channel.lvclass"=w5602:refnum<class "Channel.lvclass">, "Acquisition out"=w5603:refnum<class "Acquisition.lvclass">)  [unwired: 7 in]
                n2511 = call-dynamic "Read Interface.vi"("error in (no error)"=w5601, "Channel in"=w5602) -> ("error out"=w5553:errorcluster, "Interface.lvclass"=w5554:refnum<class "Interface.lvclass">, "Channel out"=w5547:refnum<class "Channel.lvclass">)  [unwired: 7 in]
                n2512 = call-dynamic "Write restoreExpTime.vi"("error in (no error)"=w5553, "restoreExpTime"=TRUE, "Interface in"=w5554) -> ("error out"=w5543:errorcluster, "Interface out"=w5544:refnum<class "Interface.lvclass">)  [unwired: 7 in]
                n2513 = call-dynamic "Read target cluster.vi"("error in (no error)"=w5543, "Channel in"=w5547) -> ("error out"=w5542:errorcluster, "target cluster"=w5545:T30, "Channel out"=w5546:refnum<class "Channel.lvclass">)  [unwired: 7 in]
                n2514 = stacked-sequence {
                  tunnel: [_ w5609] -> w5551
                  tunnel: w5545 -> [_ w5606]
                  tunnel: w5545 -> [w5605 _]
                  tunnel: [w5604 _] -> w5557
                  frame #0 {
                    n2515 = Unbundle By Name(w5605) -> ("FRAME_TRANSFER"=w5604:bool)
                  }
                  frame #1 {
                    # "closed"
                    n2516 = Bundle By Name(cluster=w5606, "SHUTTER_MODE"=u8 2, "FRAME_TRANSFER"=FALSE) -> (w5609:T30)
                  }
                }
                n2517 = call-dynamic "Write PREV_FT.vi"("error in (no error)"=w5542, "PREV_FT"=w5557, "Interface in"=w5544) -> ("error out"=w5548:errorcluster, "Interface out"=w5541:refnum<class "Interface.lvclass">)  [unwired: 7 in]
                n2518 = call-dynamic "Write target cluster.vi"("error in (no error)"=w5548, "target cluster"=w5551, "Channel in"=w5546) -> ("error out"=w5550:errorcluster, "Channel out"=w5549:refnum<class "Channel.lvclass">)  [unwired: 7 in]
                n2519 = Flatten To String(anything=w5551, error in (no error)=w5550) -> (data string=w5598:string, error out=w5597:errorcluster)  [unwired: 2 in, 1 out]
                n2520 = call "Write flatted cluster.vi"("error in (no error)"=w5597, "flatted cluster"=w5598, "Interface in"=w5541) -> ("error out"=w5595:errorcluster, "Interface out"=w5596:refnum<class "Interface.lvclass">)  [unwired: 7 in]
                n2521 = call-dynamic "Write Interface.vi"("error in (no error)"=w5595, "Interface.lvclass"=w5596, "Channel in"=w5549) -> ("error out"=w5591:errorcluster, "Channel out"=w5590:refnum<class "Channel.lvclass">)  [unwired: 7 in]
                n2522 = call "Write section_name.vi"("error in (no error)"=w5591, "section_name"="CCD_ACS1", "Channel in"=w5590) -> ("error out"=w5592:errorcluster, "Channel out"=w5587:refnum<class "Channel.lvclass">)  [unwired: 7 in]
                n2523 = call-dynamic "save config.vi"("error in (no error)"=w5592, "file config"="lastsaved.cfg", "Channel in"=w5587) -> ("error out"=w5571:errorcluster, "Channel out"=w5572:refnum<class "Channel.lvclass">)  [unwired: 7 in]
                n2524 = local read "Filter1"() -> (w5573:u8)
                n2525 = call-dynamic "Write Filter.vi"("error in (no error)"=w5571, "Filter"=w5573, "Channel in"=w5572) -> ("error out"=w5580:errorcluster, "Channel out"=w5570:refnum<class "Channel.lvclass">)  [unwired: 7 in]
                n2526 = call-dynamic "Read Interface.vi"("error in (no error)"=w5580, "Channel in"=w5570) -> ("error out"=w5578:errorcluster, "Interface.lvclass"=w5569:refnum<class "Interface.lvclass">, "Channel out"=w5563:refnum<class "Channel.lvclass">)  [unwired: 7 in]
                n2527 = call-dynamic "Write Suffix.vi"("error in (no error)"=w5578, "Suffix"=w5556, "Interface in"=w5569) -> ("error out"=w5574:errorcluster, "Interface out"=w5568:refnum<class "Interface.lvclass">)  [unwired: 7 in]
                n2528 = call-dynamic "Write ObsType.vi"("error in (no error)"=w5574, "ObsType"=w5555, "Interface in"=w5568) -> ("error out"=w5575:errorcluster, "Interface out"=w5567:refnum<class "Interface.lvclass">)  [unwired: 7 in]
                n2529 = call-dynamic "Write Object.vi"("error in (no error)"=w5575, "Object"=w5558, "Interface in"=w5567) -> ("error out"=w5576:errorcluster, "Interface out"=w5566:refnum<class "Interface.lvclass">)  [unwired: 7 in]
                n2530 = call-dynamic "Write Comments.vi"("error in (no error)"=w5576, "Comments"=w5559, "Interface in"=w5566) -> ("error out"=w5577:errorcluster, "Interface out"=w5565:refnum<class "Interface.lvclass">)  [unwired: 7 in]
                n2531 = call-dynamic "Write Observer.vi"("error in (no error)"=w5577, "Observer"=w5560, "Interface in"=w5565) -> ("error out"=w5579:errorcluster, "Interface out"=w5564:refnum<class "Interface.lvclass">)  [unwired: 7 in]
                n2532 = call-dynamic "Write Interface.vi"("error in (no error)"=w5579, "Interface.lvclass"=w5564, "Channel in"=w5563) -> ("error out"=w5561:errorcluster, "Channel out"=w5562:refnum<class "Channel.lvclass">)  [unwired: 7 in]
                n2533 = call-dynamic "Read State Machine.vi"("error in (no error)"=w5561, "Device in"=w5562) -> ("error out"=w5527:errorcluster, "State Machine.lvclass"=w5530:refnum<class "State Machine.lvclass">, "Device out"=w5586:refnum<class "Channel.lvclass">)  [unwired: 7 in]
                n2534 = call-dynamic "Read ref StatesQueue.vi"("error in (no error)"=w5527, "State Machine in"=w5530) -> ("error out"=w5534:errorcluster, "ref StatesQueue"=w5533:refnum<queue>, "State Machine out"=w5529:refnum<class "State Machine.lvclass">)  [unwired: 7 in]
                n2535 = Flush Queue(queue=w5533, error in (no error)=w5534) -> (queue out=w5535:refnum<queue>, error out=w5539:errorcluster)  [unwired: 1 out]
                n2536 = Enqueue Element(queue=w5535, element=u32 300 ("State"), error in (no error)=w5539) -> (queue out=w5536:refnum<queue>, error out=w5540:errorcluster)  [unwired: 1 in, 1 out]
                n2537 = Enqueue Element(queue=w5536, element=u32 60 ("State"), error in (no error)=w5540) -> (queue out=w5537:refnum<queue>, error out=w5538:errorcluster)  [unwired: 1 in, 1 out]
                n2538 = call-dynamic "Write ref StatesQueue.vi"("error in (no error)"=w5538, "ref StatesQueue"=w5537, "State Machine in"=w5529) -> ("error out"=w5526:errorcluster, "State Machine out"=w5528:refnum<class "State Machine.lvclass">)  [unwired: 7 in]
                n2539 = call-dynamic "Write State.vi"("error in (no error)"=w5526, "State"=0, "State Machine in"=w5528) -> ("error out"=w5594:errorcluster, "State Machine out"=w5585:refnum<class "State Machine.lvclass">)  [unwired: 7 in]
                n2540 = call-dynamic "Write State Machine.vi"("error in (no error)"=w5594, "State Machine.lvclass"=w5585, "Device in"=w5586) -> ("error out"=w5583:errorcluster, "Device out"=w5584:refnum<class "Channel.lvclass">)  [unwired: 7 in]
                n2541 = call-dynamic "Write Channel.vi"("error in (no error)"=w5583, "Channel.lvclass"=w5584, "Acquisition in"=w5603) -> ("error out"=w5600:errorcluster, "Acquisition out"=w5599:refnum<class "Acquisition.lvclass">)  [unwired: 7 in]
              }
            }
            n2542 = case shown="True" w5246 {
              tunnel: w5248 -> [w5353 w5412]
              tunnel: w5247 -> [w5352 w5411]
              tunnel: [w5353 w5410] -> w5261
              tunnel: [w5352 w5409] -> w5260
              tunnel: w5236 -> [_ w5388]
              tunnel: w5235 -> [_ w5387]
              tunnel: w5234 -> [_ w5386]
              tunnel: w5233 -> [_ w5384]
              tunnel: w5232 -> [_ w5383]
              frame False {
              }
              frame True {
                # "nome do arquivo .cfg"
                # "seção no arquivo .cfg"
                n2543 = call-dynamic "Read Channel.vi"("error in (no error)"=w5411, "Acquisition in"=w5412) -> ("error out"=w5415:errorcluster, "Channel.lvclass"=w5414:refnum<class "Channel.lvclass">, "Acquisition out"=w5413:refnum<class "Acquisition.lvclass">)  [unwired: 7 in]
                n2544 = call-dynamic "Read Interface.vi"("error in (no error)"=w5415, "Channel in"=w5414) -> ("error out"=w5380:errorcluster, "Interface.lvclass"=w5381:refnum<class "Interface.lvclass">, "Channel out"=w5378:refnum<class "Channel.lvclass">)  [unwired: 7 in]
                n2545 = call-dynamic "Write restoreExpTime.vi"("error in (no error)"=w5380, "restoreExpTime"=TRUE, "Interface in"=w5381) -> ("error out"=w5373:errorcluster, "Interface out"=w5379:refnum<class "Interface.lvclass">)  [unwired: 7 in]
                n2546 = call-dynamic "Read target cluster.vi"("error in (no error)"=w5373, "Channel in"=w5378) -> ("error out"=w5372:errorcluster, "target cluster"=w5374:T30, "Channel out"=w5370:refnum<class "Channel.lvclass">)  [unwired: 7 in]
                n2547 = stacked-sequence {
                  tunnel: [_ w5436] -> w5376
                  tunnel: w5374 -> [_ w5435]
                  tunnel: w5374 -> [w5433 _]
                  tunnel: [w5432 _] -> w5385
                  frame #0 {
                    n2548 = Unbundle By Name(w5433) -> ("FRAME_TRANSFER"=w5432:bool)
                  }
                  frame #1 {
                    # "closed"
                    n2549 = Bundle By Name(cluster=w5435, "SHUTTER_MODE"=u8 2, "FRAME_TRANSFER"=FALSE) -> (w5436:T30)
                  }
                }
                n2550 = call-dynamic "Write PREV_FT.vi"("error in (no error)"=w5372, "PREV_FT"=w5385, "Interface in"=w5379) -> ("error out"=w5375:errorcluster, "Interface out"=w5377:refnum<class "Interface.lvclass">)  [unwired: 7 in]
                n2551 = call-dynamic "Write target cluster.vi"("error in (no error)"=w5375, "target cluster"=w5376, "Channel in"=w5370) -> ("error out"=w5371:errorcluster, "Channel out"=w5369:refnum<class "Channel.lvclass">)  [unwired: 7 in]
                n2552 = Flatten To String(anything=w5376, error in (no error)=w5371) -> (data string=w5416:string, error out=w5417:errorcluster)  [unwired: 2 in, 1 out]
                n2553 = call "Write flatted cluster.vi"("error in (no error)"=w5417, "flatted cluster"=w5416, "Interface in"=w5377) -> ("error out"=w5419:errorcluster, "Interface out"=w5418:refnum<class "Interface.lvclass">)  [unwired: 7 in]
                n2554 = call-dynamic "Write Interface.vi"("error in (no error)"=w5419, "Interface.lvclass"=w5418, "Channel in"=w5369) -> ("error out"=w5423:errorcluster, "Channel out"=w5424:refnum<class "Channel.lvclass">)  [unwired: 7 in]
